vi "Randomize Statuses.vi"(9 "MicrogridID":u16, 10 "DeviceID":T1) -> (3 "IED Status Array out":T2[](array[typedef]))   [LabVIEW 2018, in "IED Test Framework.lvlib" / "IED Test.lvclass"]
uses:
  IED Test.lvclass
  <vilib>/ORNL/CSEISMIC DDS/CSEISMIC DDS Base/Data Types/IED_Status.ctl
  <vilib>/ORNL/CSEISMIC DDS/CSEISMIC DDS Base/Data Types/Controls/DeviceID.ctl
  <vilib>/ORNL/CSEISMIC DDS/CSEISMIC DDS Base/Data Types/Controls/Timestamp.ctl
  <vilib>/ORNL/CSEISMIC DDS/CSEISMIC DDS Base/CSEISMIC DDS.lvclass
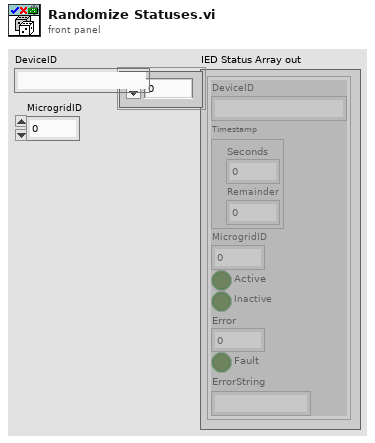
[diagram p1: front panel]
types:
  T1 = typedef "CSEISMIC DDS.lvlib/CSEISMIC DDS.lvclass/DeviceID.ctl" = string
  T2 = typedef "CSEISMIC DDS.lvlib/CSEISMIC DDS.lvclass/IED_Status.ctl" = cluster{"DeviceID":T1, "Timestamp":T3, "MicrogridID":u8, "Active":bool, "Inactive":bool, "Error":i32, "Fault":bool, "ErrorString":string}
  T3 = typedef "CSEISMIC DDS.lvlib/CSEISMIC DDS.lvclass/Timestamp.ctl" = cluster{"Seconds":u64, "Remainder":u64}
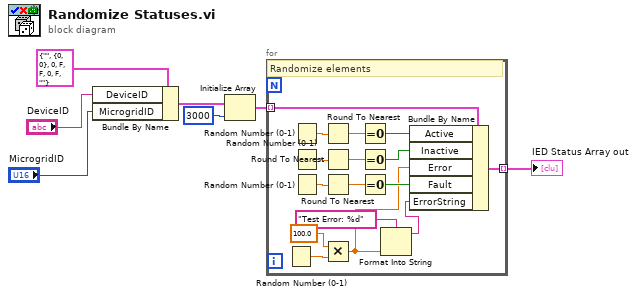
[diagram p0: block diagram]
diagram:
  n1 = Bundle By Name(cluster=T2 {"DeviceID"="", "Timestamp"={"Seconds"=0, "Remainder"=0}, "MicrogridID"=0, "Active"=FALSE, "Inactive"=FALSE, "Error"=0, "Fault"=FALSE, "ErrorString"=""} ("Status_IED"), "DeviceID"="DeviceID", "MicrogridID"="MicrogridID") -> (w6:T2)
  n2 = Initialize Array(w6, 3000 ("dimension size")) -> (w2:T2[])
  n3 = for {
    tunnel: w2 -> [w23] mode=indexing
    tunnel: [w11] -> w1 mode=indexing
    # "Randomize elements"
    n4 = Random Number (0-1)() -> (number: 0 to 1=w13:dbl)
    n5 = Random Number (0-1)() -> (number: 0 to 1=w22:dbl)
    n6 = Random Number (0-1)() -> (number: 0 to 1=w21:dbl)
    n7 = Random Number (0-1)() -> (number: 0 to 1=w20:dbl)
    n8 = Round To Nearest(number=w22) -> (nearest integer value=w19:dbl)
    n9 = Round To Nearest(number=w21) -> (nearest integer value=w18:dbl)
    n10 = Round To Nearest(number=w20) -> (nearest integer value=w17:dbl)
    n11 = Multiply(x=100.0, y=w13) -> (x*y=w10:dbl)
    n12 = Equal To 0?(x=w19) -> (x = 0?=w16:bool)
    n13 = Equal To 0?(x=w18) -> (x = 0?=w15:bool)
    n14 = Equal To 0?(x=w17) -> (x = 0?=w14:bool)
    n15 = Format Into String(format string="Test Error: %d", w10) -> (resulting string=w8:string)  [unwired: 2 in, 1 out]
    n16 = Bundle By Name(cluster=w23, "Active"=w16, "Inactive"=w15, "Error"=w10, "Fault"=w14, "ErrorString"=w8) -> (w11:T2)
  }
  "IED Status Array out" <- w1
